vi "Gen - System Config.vi"() -> (3 "Data Out":T1={"HMI Configuration"={"EXE Name"="", "Project Name"="", "Max Page No"=2, "HMI State"=enum."Maximized", "Version"=enum."Demo", "Check License"=FALSE, "Font Size"=44, "Res: Height"=655, "Res: Width"=1356, "License Level"=enum."Level 2", "License Type"=enum."Perpetual"}, "All HMI Module"=["Module - DAQmx AI Daemon.vit", "Module - DAQmx AI.vi", "Module - DAQmx AO.vi", "Module - DAQmx DI.vi", "Module - DAQmx DO.vi", "Module - Error Management.vi", "Module - Login.vi", "Module - P1 Display.vi", "Module - P2 List Device.vi", "Module - P3 Configure Tags IO.vi", "Module - P4 Log Config.vi", "Module - P5 Filter.vi", "Module - P6 Calibration.vi", "Module - P7 Analysis.vi", "Module - P8 User Management.vi"], "Default HMI Module"=["Module - Error Management.vi", "Module - Login.vi", "Module - P1 Display.vi", "Module - P2 List Device.vi", "Module - P3 Configure Tags IO.vi", "Module - P4 Log Config.vi", "Module - P5 Filter.vi", "Module - P6 Calibration.vi", "Module - P7 Analysis.vi", "Module - P8 User Management.vi"], "Page Module"=["Module - P1 Display.vi", "Module - P2 List Device.vi", "Module - P3 Configure Tags IO.vi", "Module - P4 Log Config.vi", "Module - P5 Filter.vi", "Module - P6 Calibration.vi", "Module - P7 Analysis.vi", "Module - P8 User Management.vi"], "Page List: Level 1"=[], "Page List: Level 2"=[], "Page List: Level 3"=[], "All RT Module"=[], "Default RT Module"=[], "Acquire Enable Page"=[], "Log Enable Page"=[], "Run Page"=[], "Kill Page"=[], "Button"={"Text"=["", "", "", "", "", "", "", ""], "Tip Strip"=[]}})   [LabVIEW 2020]
uses:
  Control/Page List Configuration.ctl
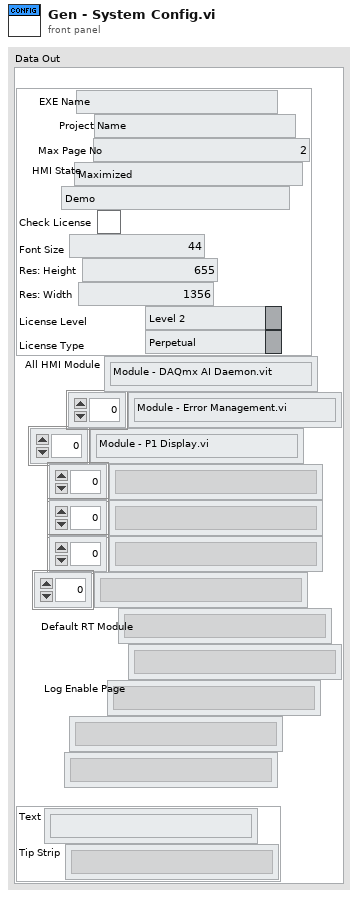
[diagram p1: front panel]
types:
  T1 = typedef "Page List Configuration.ctl" = cluster{"HMI Configuration":cluster{"EXE Name":string, "Project Name":string, "Max Page No":i32, "HMI State":enum32{"Invalid", "Standard", "Closed", "Hidden", "Minimized", "Maximized"}, "Version":enum16{"Demo", "User"}, "Check License":bool, "Font Size":u32, "Res: Height":i16, "Res: Width":i16, "License Level":enum16{"Level 1", "Level 2", "Level 3", "Level 4", "Level 5"}, "License Type":enum16{"Free", "Trial", "Subscription", "Perpetual"}}, "All HMI Module":string[], "Default HMI Module":string[], "Page Module":string[], "Page List: Level 1":string[], "Page List: Level 2":string[], "Page List: Level 3":string[], "All RT Module":string[], "Default RT Module":string[], "Acquire Enable Page":string[], "Log Enable Page":string[], "Run Page":string[], "Kill Page":string[], "Button":cluster{"Text":string[], "Tip Strip":string[]}}
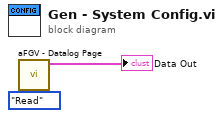
[diagram p0: block diagram]
diagram:
  n1 = call "aFGV - Datalog Page.vi"("Action"=enum16{"Read", "Write"}."Read") -> ("Data Out"=→"Data Out":T1)  [unwired: 9 in, 1 out]
